vi "Hardware_Control_From_Joystick.vi"() -> ()   [LabVIEW 2018]
uses:
  <vilib>/LabVIEW Interface for Arduino/Type Defs/Board Type.ctl
  <vilib>/LabVIEW Interface for Arduino/Type Defs/Connection Type.ctl
  <vilib>/LabVIEW Interface for Arduino/Type Defs/Pin Mode.ctl
  <vilib>/LabVIEW Interface for Arduino/LabVIEW Interface for Arduino.lvlib
panel:
  in  "Stop":bool
  out "Servo 2 FB":dbl(knob) scale=0.0..180.0
  out "Servo 1 FB":dbl(knob) scale=0.0..180.0
  in  "Com port Selection":refnum<visa-resource-name>
  in  "Arduino Board Selection":T1
  in  "Cycle start Button":bool
  in  "servo pin 2":u8=2
  in  "Number of servo":u8=1
  in  "servo pin 1":u8=2
  in  "Color Box 2":u32(colorbox)
  # "Control Panel"
  # "Instructions:\n1. Set servo pin from GUI Control elements\n2. Set arduino board type from GUI control\n3. set com port from GUI control\n4. Servo will function only when \"Cycle start button pressed\".\n5. For Joystick, analog pin 0 and 1 used respectively for X and Y axis"
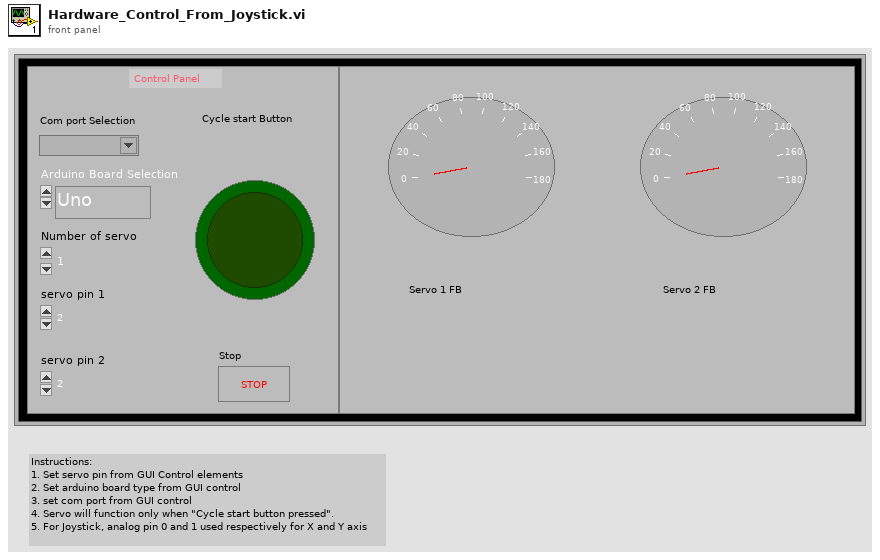
[diagram p1: front panel]
types:
  T1 = typedef "LabVIEW Interface for Arduino.lvlib/Board Type.ctl" = enum16{"Uno", "Dimuelanove w/Atmega 328", "Mega 2560"}
  T2 = typedef "LabVIEW Interface for Arduino.lvlib/Connection Type.ctl" = enum8{"USB / Serial", "XBEE", "BlueSmirf (Bluetooth)"}
  T3 = typedef "LabVIEW Interface for Arduino.lvlib/Arduino Resource.ctl" = cluster{"VISA resource":refnum<visa-resource-name>, "Board Type":T1, "Connection Type":enum8{"USB / Serial"}, "Bytes Per Packet (15)":u8}
  T4 = typedef "LabVIEW Interface for Arduino.lvlib/Pin Mode.ctl" = enum8{"Input", "Output"}
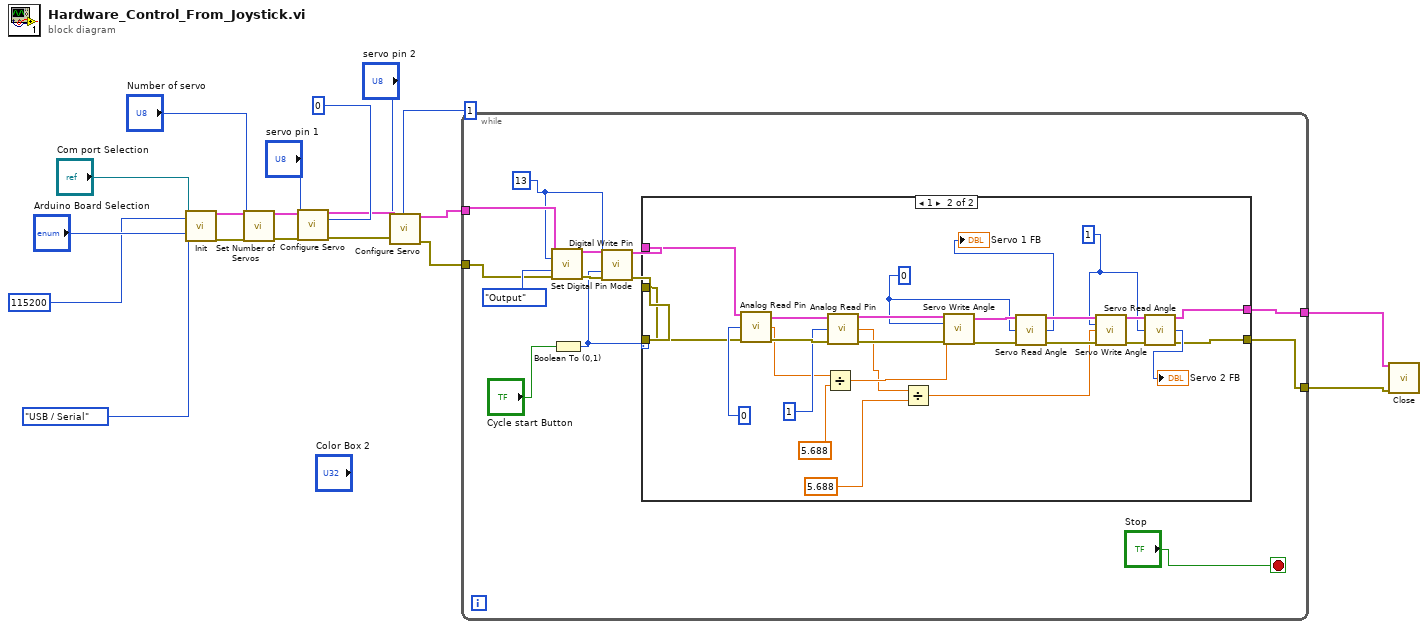
[diagram p0: block diagram]
diagram:
  n1 = call <vilib>:"Init.vi"("VISA resource"="Com port Selection", "Baud Rate (115200)"=u32 115200, "Board Type (Uno)"="Arduino Board Selection", "Connection Type (USB/Serial)"=Connection_Type."USB / Serial") -> ("Arduino Resource"=w17:T3, "error out"=w16:errorcluster)  [unwired: 14 in]
  n2 = call <vilib>:"Set Number of Servos.vi"("Arduino Resource"=w17, "Number Of Servos (1)"="Number of servo", "error in"=w16) -> ("Arduino Resource"=w14:T3, "error out"=w13:errorcluster)  [unwired: 11 in]
  n3 = call <vilib>:"Configure Servo.vi"("Arduino Resource"=w14, "Servo Number (0)"=u8 0, "DIO Pin (2)"="servo pin 1", "error in"=w13) -> ("Arduino Resource"=w10:T3, "error out"=w9:errorcluster)  [unwired: 10 in]
  n4 = call <vilib>:"Configure Servo.vi"("Arduino Resource"=w10, "Servo Number (0)"=u8 1, "DIO Pin (2)"="servo pin 2", "error in"=w9) -> ("Arduino Resource"=w6:T3, "error out"=w5:errorcluster)  [unwired: 10 in]
  n5 = while {
    tunnel: w6 -> [w31]
    tunnel: w5 -> [w27]
    tunnel: [w26] -> w4
    tunnel: [w25] -> w3
    stop <- "Stop" stop-if-true
    w24 = u8 13 ("Digital I/O Pin")
    n6 = call <vilib>:"Set Digital Pin Mode.vi"("Arduino Resource"=w31, "Digital I/O Pin"=w24, "Pin Mode (Input)"=Pin_Mode."Output", "error in"=w27) -> ("Arduino Resource"=w32:T3, "error out"=w29:errorcluster)  [unwired: 10 in]
    n7 = Boolean To (0,1)(Boolean="Cycle start Button") -> (0, 1=w22:i16)
    n8 = call <vilib>:"Digital Write Pin.vi"("Arduino Resource"=w32, "Digital I/O Pin (0)"=w24, "Value (0)"=w22, "error in"=w29) -> ("Arduino Resource"=w28:T3, "error out"=w20:errorcluster)  [unwired: 10 in]
    n9 = case shown="1" w22 {
      tunnel: w28 -> [w34 w36]
      tunnel: [w34 w40] -> w26
      tunnel: [w33 w39] -> w25
      tunnel: w20 -> [w33 _]
      tunnel: w20 -> [_ w35]
      frame 0, Default {
      }
      frame 1 {
        w38 = u8 1 ("Servo Number")
        w37 = u8 0 ("Servo Number")
        n10 = call <vilib>:"Analog Read Pin.vi"("Arduino Resource"=w36, "Analog Input Pin (0)"=u8 0, "error in"=w35) -> ("Arduino Resource"=w58:T3, "Voltage"=w48:dbl, "error out"=w57:errorcluster)  [unwired: 10 in]
        n11 = Divide(x=w48, y=5.688) -> (x/y=w46:dbl)
        n12 = call <vilib>:"Analog Read Pin.vi"("Arduino Resource"=w58, "Analog Input Pin (0)"=u8 1, "error in"=w57) -> ("Arduino Resource"=w50:T3, "Voltage"=w45:dbl, "error out"=w49:errorcluster)  [unwired: 10 in]
        n13 = Divide(x=w45, y=5.688) -> (x/y=w43:dbl)
        n14 = call <vilib>:"Servo Write Angle.vi"("Arduino Resource"=w50, "Servo Number"=w37, "Angle (Degrees)"=w46, "error in"=w49) -> ("Arduino Resource"=w54:T3, "error out"=w53:errorcluster)  [unwired: 10 in]
        n15 = call <vilib>:"Servo Read Angle.vi"("Arduino Resource"=w54, "Servo Number"=w37, "error in"=w53) -> ("Arduino Resource"=w52:T3, "Angle (Degrees)"=→"Servo 1 FB":u8, "error out"=w51:errorcluster)  [unwired: 10 in]
        n16 = call <vilib>:"Servo Write Angle.vi"("Arduino Resource"=w52, "Servo Number"=w38, "Angle (Degrees)"=w43, "error in"=w51) -> ("Arduino Resource"=w60:T3, "error out"=w59:errorcluster)  [unwired: 10 in]
        n17 = call <vilib>:"Servo Read Angle.vi"("Arduino Resource"=w60, "Servo Number"=w38, "error in"=w59) -> ("Arduino Resource"=w40:T3, "Angle (Degrees)"=→"Servo 2 FB":u8, "error out"=w39:errorcluster)  [unwired: 10 in]
      }
    }
  }
  n18 = call <vilib>:"Close.vi"("Arduino Resource"=w4, "error in"=w3) -> ()  [unwired: 13 in, 1 out]
